vi "Autonomous Independent.vi"() -> ()   [LabVIEW 2016]
doc: "This VI is called when autonomous begins, and will automatically be terminated when autonomous ends. You can carry out timed or sensor driven robot movement independently without needing to return to the caller."
uses:
  <vilib>/Rock Robotics/WPI/Utilities/WPI_GetSetVariantRefNum.vi
  <vilib>/Rock Robotics/Network Tables/NT Write Numeric Array.vi
  <vilib>/Rock Robotics/Network Tables/NT Read Boolean.vi
  <vilib>/Rock Robotics/Network Tables/NT Write Number.vi
  <vilib>/Rock Robotics/WPI/RobotDrive/WPI_RobotDriveArcadeDrive_Standard(NoSaturation).vi
  <vilib>/Rock Robotics/Network Tables/NT Write Boolean.vi
  <vilib>/Rock Robotics/Network Tables/NT Read Number.vi
panel:
  out "Left + Right OverSpeed":cluster{dbl, dbl}(knob)={10.0, -10.0} scale=-10.0..10.0
  out "Difference":dbl(knob) scale=0.0..50.0
  in  "Reset Counters":bool
  out "Right Wheel Sensor Count":dbl
  out "Left Wheel Sensor Count":dbl
  out "POT Sensor Meter 3":dbl(knob)=78.0 scale=78.0..98.0
  out "POT Sensor Value 3":dbl
  out "Frame 0 - Hit Low Sensor":bool
  out "Frame 10 - Raised to Value":bool
  out "Frame 8  - TickSensor 1":bool
  out "Frame 6  - TickSensor 1":bool
  out "Frame 4 - TickSensor 1":bool
  out "Frame 2 - TickSensor 1":bool
  in  "Ticks to Turn Right":i32
  in  "To goto the edge of the goal":i32=9
  in  "Value to Raise to.":dbl=90.0
  in  "Ticks to Turn Left":i32=9
  in  "Distance to goto pass the Defence":i32=30
  in  "Ticks to Drive forwad close to the turnning Point":i32=42
  in  "Desides the Distance for Loop 1":i32=16
  out "VAR-Storage-1":dbl
  out "Low Switch":bool
  out "High Switch":bool
  # "Also This value is the \nTotal amount of ticks not Turns!\n\nSo 6 Ticks EQU 1 Full Turn."
  # "Remeber to Right Click:\nData Operatoins -> Make Current Value Default"
  # "LOOP 1 - LOOP 1 - LOOP 1 - LOOP 1 - LOOP 1 - LOOP 1 - LOOP 1 - LOOP 1 - LOOP 1 - LOOP 1 - LOOP 1"
  # "DRIVE PAST THE DEFENCE"
  # "LOOP 2  - LOOP 2  - LOOP 2  - LOOP 2  - LOOP 2  - LOOP 2 -  LOOP 2 - LOOP 2  - LOOP 2  - LOOP 2 - LOOP 2"
  # "THIS IS TO DRIVE PAST THE DEFENCE AND TRY TO SHOT"
  # "Left"
  # "Right"
  # "LOOP 3  - LOOP 3  - LOOP 3  - LOOP 3  - LOOP 3  - LOOP 3  - LOOP 3  - LOOP 3  - LOOP 3  - LOOP 3 - LOOP 3"
  # "Go Past the Defence."
  # "Be sure to right-click and choose Data Operations>>Make Current Value default if you want to save the array values with the VI"
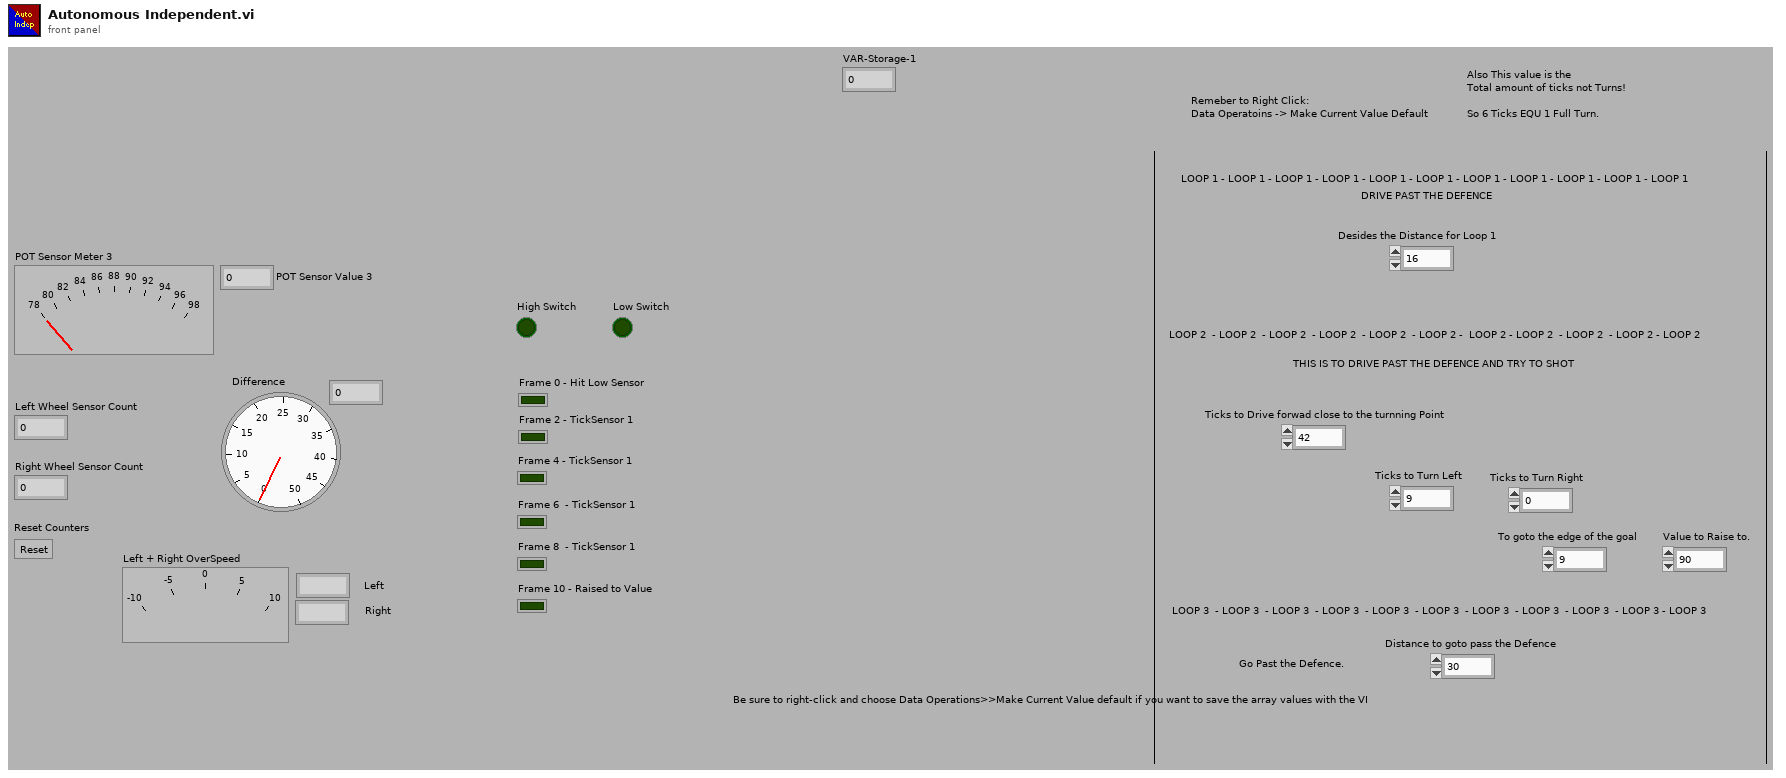
[diagram p1: front panel]
types:
  T1 = typedef "WPI_JoystickDevRef.ctl" = cluster{"Device":T2}
  T2 = typedef "WPI_JoystickDeviceEnum.ctl" = enum16{"USB 0", "USB 1", "USB 2", "USB 3", "USB 4", "USB 5"}
  T3 = typedef "WPI_RobotDriveDevRef.ctl" = cluster{"DevStatus":errorcluster, "Motors[]":T4[], "Square Inputs":bool, "Max Output":dbl}
  T4 = typedef "WPI_MotorControlDeviceRef.ctl" = cluster{"DeviceStatus":errorcluster, "Type":T5, "PWM":cluster{"PWM Channel":T6, "DeadBand":T7}, "CAN":cluster{"Device Number":u8, "SetOutput VI Ref":variant, "GetOutput VI Ref":variant, "Enable VI Ref":variant, "Disable VI Ref":variant, "Data":variant}, "Invert":bool}
  T5 = typedef "WPI_MotorControlType.ctl" = enum16{"PWM", "CAN"}
  T6 = typedef "FPGA_DIOPWMChannel.ctl" = enum8{"PWM 0", "PWM 1", "PWM 2", "PWM 3", "PWM 4", "PWM 5", "PWM 6", "PWM 7", "PWM 8", "PWM 9", "PWM MXP 0", "PWM MXP 1", "PWM MXP 2", "PWM MXP 3", "PWM MXP 4", "PWM MXP 5", "PWM MXP 6", "PWM MXP 7", "PWM MXP 8", "PWM MXP 9", "Invalid"}
  T7 = typedef "WPI_PWMDeadband.ctl" = cluster{"Name":string, "maxPositivePwm":i32, "minPositivePwm":i32, "centerPwm":i32, "maxNegativePwm":i32, "minNegativePwm":i32, "angularRange":u16}
  T8 = typedef "WPI_CounterDevRef.ctl" = cluster{"DevStatus":errorcluster, "CntIndex":T9}
  T9 = typedef "FPGA_CounterCtrSystemIndex.ctl" = enum8{"Ctr 0", "Ctr 1", "Ctr 2", "Ctr 3", "Ctr 4", "Ctr 5", "Ctr 6", "Ctr 7", "Invalid"}
  T10 = typedef "WPI_SwitchDevRef.ctl" = cluster{"DevStatus":errorcluster, "DIO Channel":T11, "CntIndex":T9, "Normally Closed":bool}
  T11 = typedef "FPGA_DIOChannel.ctl" = enum8{"DIO 0", "DIO 1", "DIO 2", "DIO 3", "DIO 4", "DIO 5", "DIO 6", "DIO 7", "DIO 8", "DIO 9", "DIO MXP 0", "DIO MXP 1", "DIO MXP 2", "DIO MXP 3", "DIO MXP 4", "DIO MXP 5", "DIO MXP 6", "DIO MXP 7", "DIO MXP 8", "DIO MXP 9", "DIO MXP 10", "DIO MXP 11", "DIO MXP 12", "DIO MXP 13", "DIO MXP 14", "DIO MXP 15", "SPI Port CS1", "SPI Port CS2", "SPI Port CS3", "SPI Port MISO", "SPI Port MOSI", "Invalid"}
  T12 = typedef "WPI_PotentiometerDevRef.ctl" = cluster{"DevStatus":errorcluster, "Analog Channel":T13, "Invert Output":bool}
  T13 = typedef "FPGA_AIChannel.ctl" = enum8{"AI 0", "AI 1", "AI 2", "AI 3", "AI MXP 0", "AI MXP 1", "AI MXP 2", "AI MXP 3", "Invalid"}
  T14 = typedef "WPI_ServoDeviceRef.ctl" = cluster{"DeviceStatus":errorcluster, "PWM Channel":T6, "DeadBand":T7}
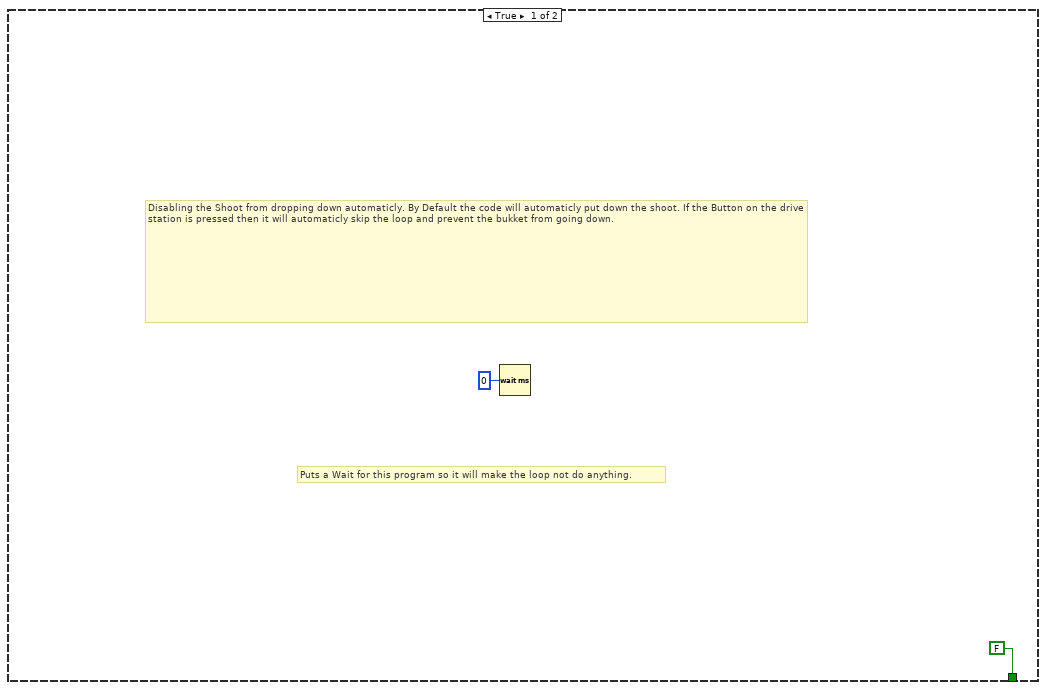
[diagram p3: hidden frame]
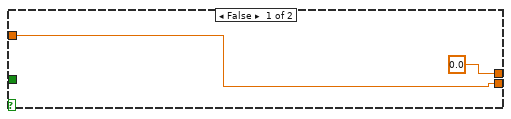
[diagram p4: hidden frame]
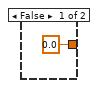
[diagram p5: hidden frame]
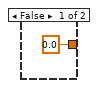
[diagram p7: hidden frame]
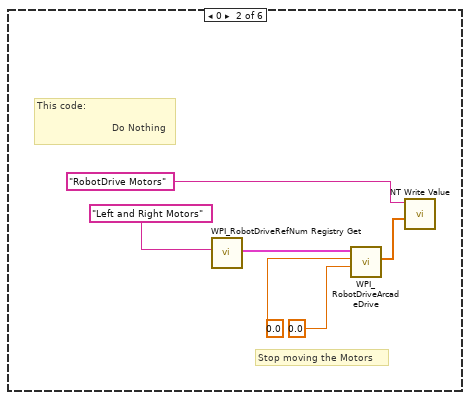
[diagram p10: hidden frame]
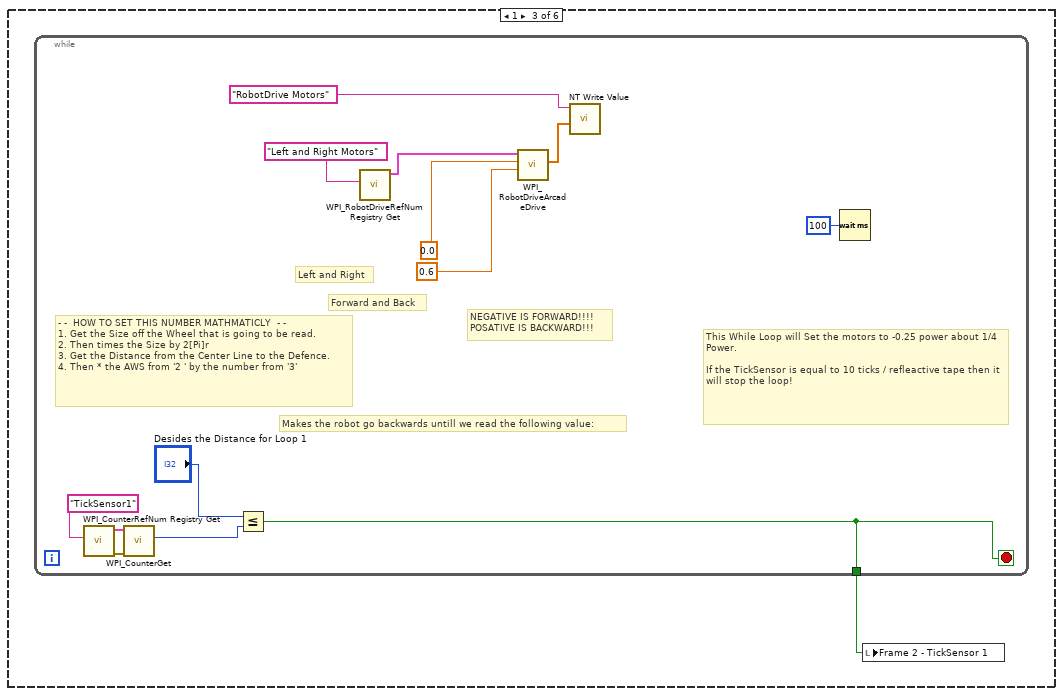
[diagram p11: hidden frame]
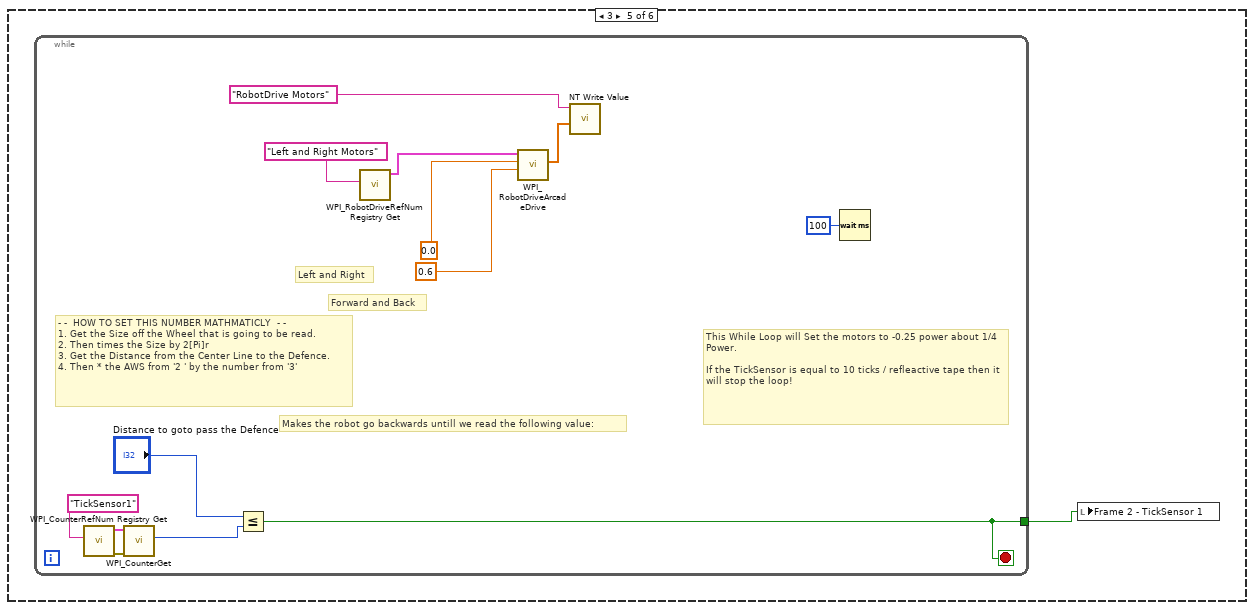
[diagram p12: hidden frame]
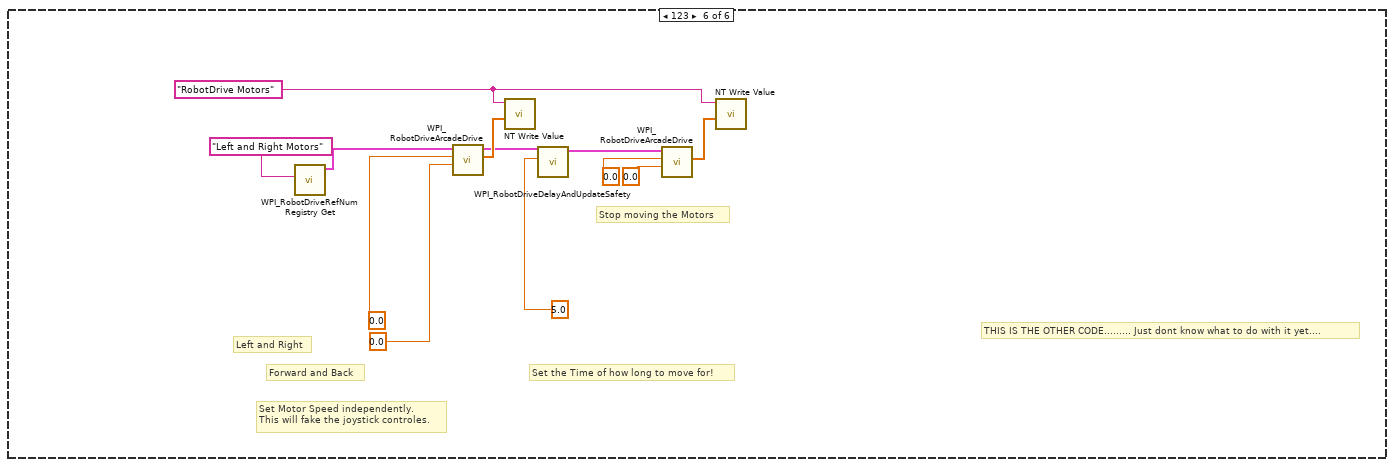
[diagram p13: hidden frame]
diagram:
  (unwired) "This function is run in parallel when the autonomous period begins. It will be terminated automatically when the period ends.\n\nNote that all Driver Station inputs are automatically latched and will not change once auto begins."
  # "Auto Count of Wheel"
  # "Every 20ms, report that we are running autonomous\ncode. Loop will abort the same time as the VI."
  # "This gives you the joystick value\nthat is often the throttle"
  # "This tells you the driver position\nand alliance color"
  n1 = call-poly <vilib>:"NT Read Value.vi"("Name"="Auto Selector") -> ()  [unwired: 9 in, 2 out]
  n2 = while {
    stop <- FALSE stop-if-true
    n3 = call <vilib>:"WPI_DriverStationReport Robot Code State.vi"("Autonomous"=TRUE) -> ()  [unwired: 10 in, 1 out]
    n4 = Wait (ms)(milliseconds to wait=u32 20) -> ()  [unwired: 1 out]
  }
  n5 = call <vilib>:"WPI_JoystickRefNum Registry Get.vi"("refnum name"="Joystick 0") -> ("JoystickDevRef"=w24:T1)  [unwired: 1 in, 9 out]
  n6 = call <vilib>:"WPI_JoystickGetValues.vi"("JoystickDevRef"=w24) -> ("Axes"=w22:dbl[])  [unwired: 6 in, 4 out]
  n7 = call <vilib>:"WPI_DriverStationGet Alliance Info.vi"() -> ()  [unwired: 12 out]
  n8 = call-poly <vilib>:"NT Write Value.vi"("Numeric Array"=w22, "Name"="Joystick 0/Axes") -> ()  [unwired: 9 in, 1 out]
  n9 = Index Array(array=w22, index=2) -> ()  [unwired: 1 out]
  n10 = flat-sequence {
    frame #0 {
      n11 = call <vilib>:"WPI_RobotDriveRefNum Registry Get.vi"("refnum name"="Left and Right Motors") -> ("RobotDriveDevRef"=w36:T3)  [unwired: 1 in, 9 out]
      n12 = call <vilib>:"WPI_MotorControlRefNum Registry Get.vi"("refnum name"="BPMs") -> ("error out"=w31:errorcluster, "MotorControlDevRef"=w30:T4)  [unwired: 9 in]
      n13 = call <vilib>:"WPI_CounterRefNum Registry Get.vi"("refnum name"="TickSensor1") -> ("error out"=w34:errorcluster, "CounterDevRef"=w35:T8)  [unwired: 9 in]
      n14 = call <vilib>:"WPI_CounterRefNum Registry Get.vi"("refnum name"="TickSensor2") -> ("error out"=w43:errorcluster, "CounterDevRef"=w42:T8)  [unwired: 9 in]
      n15 = call <vilib>:"WPI_CounterReset.vi"("error in (no error)"=w34, "CounterDevRef in"=w35) -> ()  [unwired: 8 in, 2 out]
      n16 = call <vilib>:"WPI_CounterReset.vi"("error in (no error)"=w43, "CounterDevRef in"=w42) -> ()  [unwired: 8 in, 2 out]
      n17 = call <vilib>:"WPI_MotorControlSetOutput.vi"("error in (no error)"=w31, "Output"=0.0, "MotorControlDevRef"=w30) -> ()  [unwired: 6 in, 3 out]
      n18 = call-poly <vilib>:"WPI_RobotDriveArcadeDrive.vi"("Y axis value"=0.0 ("X axis value"), "X axis value"=0.0, "RobotDriveDevRef"=w36) -> ("Motor Values"=w38:dbl[])  [unwired: 1 in, 7 out]
      n19 = call-poly <vilib>:"NT Write Value.vi"("Numeric Array"=w38, "Name"="RobotDrive Motors") -> ()  [unwired: 9 in, 1 out]
    }
    frame #1 {
      n20 = call-poly <vilib>:"NT Read Value.vi"("Default Value"=FALSE, "Name"="DisableLowerOnStart") -> ()  [unwired: 8 in, 2 out]
      n21 = case shown="False" FALSE {
        tunnel: [FALSE w51] -> w45
        frame True {
          # "Puts a Wait for this program so it will make the loop not do anything."
          # "Disabling the Shoot from dropping down automaticly. By Default the code will automaticly put down the shoot. If the Button on the drive station is pressed then it will automaticly skip the loop and prevent the bukket from going down."
          n22 = Wait (ms)(milliseconds to wait=u32 0) -> ()  [unwired: 1 out]
        }
        frame False {
          n23 = while {
            tunnel: [w52] -> w51
            stop <- w52 stop-if-true
            n24 = call <vilib>:"WPI_SwitchRefNum Registry Get.vi"("refnum name"="LowSwitch") -> ("error out"=w69:errorcluster, "SwitchDevRef"=w70:T10)  [unwired: 9 in]
            n25 = call <vilib>:"WPI_SwitchRefNum Registry Get.vi"("refnum name"="HighSwitch") -> ("error out"=w66:errorcluster, "SwitchDevRef"=w67:T10)  [unwired: 9 in]
            n26 = call <vilib>:"WPI_SwitchGetLimitValue.vi"("error in (no error)"=w69, "SwitchDevRef"=w70) -> ("Switch Pressed"=w58:bool)  [unwired: 7 in, 2 out]
            "Low Switch" <- w58
            n27 = call <vilib>:"WPI_SwitchGetLimitValue.vi"("error in (no error)"=w66, "SwitchDevRef"=w67) -> ("Switch Pressed"=w57:bool)  [unwired: 7 in, 2 out]
            "High Switch" <- w57
            n28 = call-poly <vilib>:"NT Write Value.vi"("Boolean"=w58, "Name"="Low Sensor") -> ()  [unwired: 9 in, 1 out]
            n29 = call-poly <vilib>:"NT Write Value.vi"("Boolean"=w57, "Name"="High Sensor") -> ()  [unwired: 9 in, 1 out]
            n30 = Or(x=w58, y=w57) -> (x .or. y?=w71:bool)
            n31 = case shown="True" w71 {
              tunnel: w58 -> [_ w76]
              tunnel: w57 -> [_ w78]
              tunnel: -0.5 ("Axes[1]") -> [w72 w77]
              tunnel: [0.0 ("Axes[1]") w75] -> w60
              tunnel: [w72 w74] -> w59
              frame False {
              }
              frame True {
                n32 = case shown="True" w76 {
                  tunnel: w77 -> [_ w88]
                  tunnel: [0.0 ("Axes[1]") w87] -> w75
                  frame False {
                  }
                  frame True {
                    n33 = Greater?(x=w88, y=0.0) -> (0:w89:bool)
                    n34 = case shown="False" w89 {
                      tunnel: [0.0 ("Axes[1]") w92] -> w87
                      tunnel: w88 -> [_ w92]
                      frame False {
                        # "NO VALUE SENT"
                      }
                      frame True {
                      }
                    }
                  }
                }
                n35 = case shown="True" w78 {
                  tunnel: w77 -> [_ w80]
                  tunnel: [0.0 ("Axes[1]") w81] -> w74
                  frame False {
                  }
                  frame True {
                    n36 = Less?(x=w80, y=0.0) -> (x < y?=w82:bool)
                    n37 = case shown="False" w82 {
                      tunnel: [0.0 ("Axes[1]") w85] -> w81
                      tunnel: w80 -> [_ w85]
                      frame False {
                        # "NO VALUE SENT"
                      }
                      frame True {
                      }
                    }
                  }
                }
              }
            }
            n38 = Add(x=w60, y=w59) -> (x+y=w61:dbl)
            n39 = call <vilib>:"WPI_MotorControlRefNum Registry Get.vi"("refnum name"="Pickup Motor") -> ("error out"=w64:errorcluster, "MotorControlDevRef"=w63:T4)  [unwired: 9 in]
            n40 = local read "Low Switch"() -> (w52:bool)
            n41 = call <vilib>:"WPI_MotorControlSetOutput.vi"("error in (no error)"=w64, "Output"=w61, "MotorControlDevRef"=w63) -> ()  [unwired: 6 in, 3 out]
            n42 = Wait (ms)(milliseconds to wait=u32 100) -> ()  [unwired: 1 out]
          }
        }
      }
      "Frame 0 - Hit Low Sensor" <- w45
    }
    frame #2 {
      # "This tells you the autonomous selected\nfrom the dashboard"
      n43 = call-poly <vilib>:"NT Read Value.vi"("Name"="AutoModeSelector") -> ("Numeric"=w94:dbl)  [unwired: 9 in, 1 out]
      n44 = Wait (ms)(milliseconds to wait=u32 20) -> ()  [unwired: 1 out]
      n45 = case shown="2" w94 {
        frame Default {
          # "You can put your main auto here, or you can right-click on the case and make any\nother frame be the default case."
          # "This is the frame that will execute if no selection is made, or if it is not recognized"
        }
        frame 0 {
          # "Stop moving the Motors"
          # "This code:\n                   \n                         Do Nothing"
          n46 = call <vilib>:"WPI_RobotDriveRefNum Registry Get.vi"("refnum name"="Left and Right Motors") -> ("RobotDriveDevRef"=w96:T3)  [unwired: 1 in, 9 out]
          n47 = call-poly <vilib>:"WPI_RobotDriveArcadeDrive.vi"("Y axis value"=0.0 ("X axis value"), "X axis value"=0.0, "RobotDriveDevRef"=w96) -> ("Motor Values"=w100:dbl[])  [unwired: 1 in, 7 out]
          n48 = call-poly <vilib>:"NT Write Value.vi"("Numeric Array"=w100, "Name"="RobotDrive Motors") -> ()  [unwired: 9 in, 1 out]
        }
        frame 1 {
          n49 = while {
            tunnel: [w103] -> w102
            stop <- w103 stop-if-true
            # "NEGATIVE IS FORWARD!!!!\nPOSATIVE IS BACKWARD!!!"
            # "- -  HOW TO SET THIS NUMBER MATHMATICLY  - - \n1. Get the Size off the Wheel that is going to be read.\n2. Then times the Size by 2[Pi]r\n3. Get the Distance from the Center Line to the Defence.\n4. Then * the AWS from '2 ' by the number from '3'"
            # "Makes the robot go backwards untill we read the following value:"
            # "This While Loop will Set the motors to -0.25 power about 1/4 Power.\n\nIf the TickSensor is equal to 10 ticks / refleactive tape then it will stop the loop!"
            # "Forward and Back"
            # "Left and Right"
            n50 = call <vilib>:"WPI_CounterRefNum Registry Get.vi"("refnum name"="TickSensor1") -> ("error out"=w114:errorcluster, "CounterDevRef"=w113:T8)  [unwired: 9 in]
            n51 = call <vilib>:"WPI_CounterGet.vi"("error in (no error)"=w114, "CounterDevRef in"=w113) -> ("Value"=w105:i32)  [unwired: 4 in, 5 out]
            n52 = Less Or Equal?(x="Desides the Distance for Loop 1", y=w105) -> (x <= y?=w103:bool)
            n53 = call <vilib>:"WPI_RobotDriveRefNum Registry Get.vi"("refnum name"="Left and Right Motors") -> ("RobotDriveDevRef"=w112:T3)  [unwired: 1 in, 9 out]
            n54 = call-poly <vilib>:"WPI_RobotDriveArcadeDrive.vi"("Y axis value"=0.6 ("X axis value"), "X axis value"=0.0, "RobotDriveDevRef"=w112) -> ("Motor Values"=w110:dbl[])  [unwired: 1 in, 7 out]
            n55 = call-poly <vilib>:"NT Write Value.vi"("Numeric Array"=w110, "Name"="RobotDrive Motors") -> ()  [unwired: 9 in, 1 out]
            n56 = Wait (ms)(milliseconds to wait=u32 100) -> ()  [unwired: 1 out]
          }
          n57 = local write "Frame 2 - TickSensor 1"(w102) -> ()
        }
        frame 2 {
          n58 = flat-sequence {
            frame #0 {
              n59 = while {
                tunnel: [w117] -> w116
                stop <- w117 stop-if-true
                # "- -  HOW TO SET THIS NUMBER MATHMATICLY  - - \n1. Get the Size off the Wheel that is going to be read.\n2. Then times the Size by 2[Pi]r\n3. Get the Distance from the Center Line to the Defence.\n4. Then * the AWS from '2 ' by the number from '3'"
                # "Makes the robot go backwards untill we read the following value:"
                # "This While Loop will Set the motors to -0.25 power about 1/4 Power.\n\nIf the TickSensor is equal to 10 ticks / refleactive tape then it will stop the loop!"
                # "Forward and Back"
                # "Left and Right"
                n60 = call <vilib>:"WPI_CounterRefNum Registry Get.vi"("refnum name"="TickSensor1") -> ("error out"=w128:errorcluster, "CounterDevRef"=w127:T8)  [unwired: 9 in]
                n61 = Wait (ms)(milliseconds to wait=u32 100) -> ()  [unwired: 1 out]
                n62 = call <vilib>:"WPI_CounterGet.vi"("error in (no error)"=w128, "CounterDevRef in"=w127) -> ("Value"=w119:i32)  [unwired: 4 in, 5 out]
                n63 = Less Or Equal?(x="Ticks to Drive forwad close to the turnning Point", y=w119) -> (x <= y?=w117:bool)
                n64 = call <vilib>:"WPI_RobotDriveRefNum Registry Get.vi"("refnum name"="Left and Right Motors") -> ("RobotDriveDevRef"=w126:T3)  [unwired: 1 in, 9 out]
                n65 = call-poly <vilib>:"WPI_RobotDriveArcadeDrive.vi"("Y axis value"=0.6 ("X axis value"), "X axis value"=0.0, "RobotDriveDevRef"=w126) -> ("Motor Values"=w124:dbl[])  [unwired: 1 in, 7 out]
                n66 = call-poly <vilib>:"NT Write Value.vi"("Numeric Array"=w124, "Name"="RobotDrive Motors") -> ()  [unwired: 9 in, 1 out]
              }
              "Frame 2 - TickSensor 1" <- w116
            }
            frame #1 {
              n67 = call <vilib>:"WPI_CounterRefNum Registry Get.vi"("refnum name"="TickSensor2") -> ("error out"=w137:errorcluster, "CounterDevRef"=w136:T8)  [unwired: 9 in]
              n68 = call <vilib>:"WPI_RobotDriveRefNum Registry Get.vi"("refnum name"="Left and Right Motors") -> ("RobotDriveDevRef"=w135:T3)  [unwired: 1 in, 9 out]
              n69 = call-poly <vilib>:"WPI_RobotDriveArcadeDrive.vi"("Y axis value"=0.0 ("X axis value"), "X axis value"=0.0, "RobotDriveDevRef"=w135) -> ("Motor Values"=w133:dbl[])  [unwired: 1 in, 7 out]
              n70 = call <vilib>:"WPI_CounterRefNum Registry Get.vi"("refnum name"="TickSensor1") -> ("error out"=w140:errorcluster, "CounterDevRef"=w139:T8)  [unwired: 9 in]
              n71 = call <vilib>:"WPI_CounterReset.vi"("error in (no error)"=w137, "CounterDevRef in"=w136) -> ()  [unwired: 8 in, 2 out]
              n72 = call <vilib>:"WPI_CounterReset.vi"("error in (no error)"=w140, "CounterDevRef in"=w139) -> ()  [unwired: 8 in, 2 out]
              n73 = call-poly <vilib>:"NT Write Value.vi"("Numeric Array"=w133, "Name"="RobotDrive Motors") -> ()  [unwired: 9 in, 1 out]
            }
            frame #2 {
              n74 = while {
                tunnel: [w144] -> w142
                stop <- w144 stop-if-true
                # "Forward and Back"
                # "Left and Right"
                n75 = call <vilib>:"WPI_CounterRefNum Registry Get.vi"("refnum name"="TickSensor1") -> ("error out"=w154:errorcluster, "CounterDevRef"=w153:T8)  [unwired: 9 in]
                n76 = call <vilib>:"WPI_CounterGet.vi"("error in (no error)"=w154, "CounterDevRef in"=w153) -> ("Value"=w147:i32)  [unwired: 4 in, 5 out]
                n77 = call <vilib>:"WPI_RobotDriveRefNum Registry Get.vi"("refnum name"="Left and Right Motors") -> ("RobotDriveDevRef"=w152:T3)  [unwired: 1 in, 9 out]
                n78 = Less Or Equal?(x="Ticks to Turn Left", y=w147) -> (x <= y?=w144:bool)
                n79 = call-poly <vilib>:"WPI_RobotDriveArcadeDrive.vi"("Y axis value"=0.0 ("X axis value"), "X axis value"=-0.5, "RobotDriveDevRef"=w152) -> ("Motor Values"=w151:dbl[])  [unwired: 1 in, 7 out]
                n80 = call-poly <vilib>:"NT Write Value.vi"("Numeric Array"=w151, "Name"="RobotDrive Motors") -> ()  [unwired: 9 in, 1 out]
              }
              "Frame 4 - TickSensor 1" <- w142
              n81 = Wait (ms)(milliseconds to wait=u32 100) -> ()  [unwired: 1 out]
            }
            frame #3 {
              n82 = call <vilib>:"WPI_RobotDriveRefNum Registry Get.vi"("refnum name"="Left and Right Motors") -> ("RobotDriveDevRef"=w156:T3)  [unwired: 1 in, 9 out]
              n83 = call-poly <vilib>:"WPI_RobotDriveArcadeDrive.vi"("Y axis value"=0.0 ("X axis value"), "X axis value"=0.0, "RobotDriveDevRef"=w156) -> ("Motor Values"=w158:dbl[])  [unwired: 1 in, 7 out]
              n84 = call-poly <vilib>:"NT Write Value.vi"("Numeric Array"=w158, "Name"="RobotDrive Motors") -> ()  [unwired: 9 in, 1 out]
            }
            frame #4 {
              n85 = while {
                tunnel: [w164] -> w162
                stop <- w164 stop-if-true
                # "Forward and Back"
                # "Left and Right"
                n86 = call <vilib>:"WPI_CounterRefNum Registry Get.vi"("refnum name"="TickSensor2") -> ("error out"=w174:errorcluster, "CounterDevRef"=w173:T8)  [unwired: 9 in]
                n87 = call <vilib>:"WPI_RobotDriveRefNum Registry Get.vi"("refnum name"="Left and Right Motors") -> ("RobotDriveDevRef"=w172:T3)  [unwired: 1 in, 9 out]
                n88 = call <vilib>:"WPI_CounterGet.vi"("error in (no error)"=w174, "CounterDevRef in"=w173) -> ("Value"=w167:i32)  [unwired: 4 in, 5 out]
                n89 = call-poly <vilib>:"WPI_RobotDriveArcadeDrive.vi"("Y axis value"=0.0 ("X axis value"), "X axis value"=0.5, "RobotDriveDevRef"=w172) -> ("Motor Values"=w171:dbl[])  [unwired: 1 in, 7 out]
                n90 = Less Or Equal?(x="Ticks to Turn Right", y=w167) -> (x <= y?=w164:bool)
                n91 = call-poly <vilib>:"NT Write Value.vi"("Numeric Array"=w171, "Name"="RobotDrive Motors") -> ()  [unwired: 9 in, 1 out]
              }
              "Frame 6  - TickSensor 1" <- w162
              n92 = Wait (ms)(milliseconds to wait=u32 100) -> ()  [unwired: 1 out]
            }
            frame #5 {
              n93 = call <vilib>:"WPI_CounterRefNum Registry Get.vi"("refnum name"="TickSensor2") -> ("error out"=w183:errorcluster, "CounterDevRef"=w182:T8)  [unwired: 9 in]
              n94 = call <vilib>:"WPI_CounterRefNum Registry Get.vi"("refnum name"="TickSensor1") -> ("error out"=w186:errorcluster, "CounterDevRef"=w185:T8)  [unwired: 9 in]
              n95 = call <vilib>:"WPI_RobotDriveRefNum Registry Get.vi"("refnum name"="Left and Right Motors") -> ("RobotDriveDevRef"=w181:T3)  [unwired: 1 in, 9 out]
              n96 = call-poly <vilib>:"WPI_RobotDriveArcadeDrive.vi"("Y axis value"=0.0 ("X axis value"), "X axis value"=0.0, "RobotDriveDevRef"=w181) -> ("Motor Values"=w179:dbl[])  [unwired: 1 in, 7 out]
              n97 = call <vilib>:"WPI_CounterReset.vi"("error in (no error)"=w183, "CounterDevRef in"=w182) -> ()  [unwired: 8 in, 2 out]
              n98 = call <vilib>:"WPI_CounterReset.vi"("error in (no error)"=w186, "CounterDevRef in"=w185) -> ()  [unwired: 8 in, 2 out]
              n99 = call-poly <vilib>:"NT Write Value.vi"("Numeric Array"=w179, "Name"="RobotDrive Motors") -> ()  [unwired: 9 in, 1 out]
            }
            frame #6 {
              n100 = while {
                tunnel: [w189] -> w188
                stop <- w189 stop-if-true
                # "- -  HOW TO SET THIS NUMBER MATHMATICLY  - - \n1. Get the Size off the Wheel that is going to be read.\n2. Then times the Size by 2[Pi]r\n3. Get the Distance from the Center Line to the Defence.\n4. Then * the AWS from '2 ' by the number from '3'"
                # "Makes the robot go backwards untill we read the following value:"
                # "This While Loop will Set the motors to -0.25 power about 1/4 Power.\n\nIf the TickSensor is equal to 10 ticks / refleactive tape then it will stop the loop!"
                # "Forward and Back"
                # "Left and Right"
                n101 = call <vilib>:"WPI_CounterRefNum Registry Get.vi"("refnum name"="TickSensor1") -> ("error out"=w200:errorcluster, "CounterDevRef"=w199:T8)  [unwired: 9 in]
                n102 = Wait (ms)(milliseconds to wait=u32 100) -> ()  [unwired: 1 out]
                n103 = call <vilib>:"WPI_CounterGet.vi"("error in (no error)"=w200, "CounterDevRef in"=w199) -> ("Value"=w191:i32)  [unwired: 4 in, 5 out]
                n104 = Less Or Equal?(x="To goto the edge of the goal", y=w191) -> (x <= y?=w189:bool)
                n105 = call <vilib>:"WPI_RobotDriveRefNum Registry Get.vi"("refnum name"="Left and Right Motors") -> ("RobotDriveDevRef"=w198:T3)  [unwired: 1 in, 9 out]
                n106 = call-poly <vilib>:"WPI_RobotDriveArcadeDrive.vi"("Y axis value"=-0.6 ("X axis value"), "X axis value"=0.0, "RobotDriveDevRef"=w198) -> ("Motor Values"=w196:dbl[])  [unwired: 1 in, 7 out]
                n107 = call-poly <vilib>:"NT Write Value.vi"("Numeric Array"=w196, "Name"="RobotDrive Motors") -> ()  [unwired: 9 in, 1 out]
              }
              "Frame 8  - TickSensor 1" <- w188
            }
            frame #7 {
              n108 = call <vilib>:"WPI_CounterRefNum Registry Get.vi"("refnum name"="TickSensor2") -> ("error out"=w209:errorcluster, "CounterDevRef"=w208:T8)  [unwired: 9 in]
              n109 = call <vilib>:"WPI_CounterRefNum Registry Get.vi"("refnum name"="TickSensor1") -> ("error out"=w212:errorcluster, "CounterDevRef"=w211:T8)  [unwired: 9 in]
              n110 = call <vilib>:"WPI_CounterReset.vi"("error in (no error)"=w209, "CounterDevRef in"=w208) -> ()  [unwired: 8 in, 2 out]
              n111 = call <vilib>:"WPI_CounterReset.vi"("error in (no error)"=w212, "CounterDevRef in"=w211) -> ()  [unwired: 8 in, 2 out]
              n112 = call <vilib>:"WPI_RobotDriveRefNum Registry Get.vi"("refnum name"="Left and Right Motors") -> ("RobotDriveDevRef"=w207:T3)  [unwired: 1 in, 9 out]
              n113 = call-poly <vilib>:"WPI_RobotDriveArcadeDrive.vi"("Y axis value"=0.0 ("X axis value"), "X axis value"=0.0, "RobotDriveDevRef"=w207) -> ("Motor Values"=w205:dbl[])  [unwired: 1 in, 7 out]
              n114 = call-poly <vilib>:"NT Write Value.vi"("Numeric Array"=w205, "Name"="RobotDrive Motors") -> ()  [unwired: 9 in, 1 out]
            }
            frame #8 {
              n115 = call "Time Delay"("Delay Time (s)"=1.0) -> ()  [unwired: 10 in, 1 out]
            }
            frame #9 {
              n116 = while {
                tunnel: [w216] -> w215
                stop <- w216 stop-if-true
                # "This value will set the pickup motors to lift them up."
                # "This value will be the P.O.T. value. This will stop the Loop from running."
                n117 = call <vilib>:"WPI_PotentiometerRefNum Registry Get.vi"("refnum name"="POT Sensor") -> ("error out"=w228:errorcluster, "PotDevRef"=w227:T12)  [unwired: 9 in]
                n118 = call <vilib>:"WPI_PotentiometerGetNormalized.vi"("error in"=w228, "PotDevRef"=w227) -> ("Normalized Value"=w225:dbl)  [unwired: 7 in, 2 out]
                n119 = Multiply(x=w225, y=100.0) -> (x*y=w223:dbl)
                n120 = call <vilib>:"WPI_MotorControlRefNum Registry Get.vi"("refnum name"="Pickup Motor") -> ("error out"=w222:errorcluster, "MotorControlDevRef"=w221:T4)  [unwired: 9 in]
                n121 = Less Or Equal?(x=w223, y="Value to Raise to.") -> (x <= y?=w216:bool)
                n122 = call <vilib>:"WPI_MotorControlSetOutput.vi"("error in (no error)"=w222, "Output"=0.6, "MotorControlDevRef"=w221) -> ()  [unwired: 6 in, 3 out]
                n123 = Wait (ms)(milliseconds to wait=u32 100) -> ()  [unwired: 1 out]
              }
              "Frame 10 - Raised to Value" <- w215
            }
            frame #10 {
              n124 = call <vilib>:"WPI_MotorControlRefNum Registry Get.vi"("refnum name"="BPMs") -> ("error out"=w235:errorcluster, "MotorControlDevRef"=w234:T4)  [unwired: 9 in]
              n125 = call <vilib>:"WPI_MotorControlRefNum Registry Get.vi"("refnum name"="Pickup Motor") -> ("error out"=w231:errorcluster, "MotorControlDevRef"=w230:T4)  [unwired: 9 in]
              n126 = call <vilib>:"WPI_MotorControlSetOutput.vi"("error in (no error)"=w235, "Output"=0.0, "MotorControlDevRef"=w234) -> ()  [unwired: 6 in, 3 out]
              n127 = call <vilib>:"WPI_MotorControlSetOutput.vi"("error in (no error)"=w231, "Output"=0.0, "MotorControlDevRef"=w230) -> ()  [unwired: 6 in, 3 out]
            }
            frame #11 {
              n128 = call "Time Delay3"("Delay Time (s)"=0.5) -> ()  [unwired: 10 in, 1 out]
            }
            frame #12 {
              n129 = call <vilib>:"WPI_MotorControlRefNum Registry Get.vi"("refnum name"="BPMs") -> ("error out"=w240:errorcluster, "MotorControlDevRef"=w239:T4)  [unwired: 9 in]
              n130 = call <vilib>:"WPI_MotorControlSetOutput.vi"("error in (no error)"=w240, "Output"=-0.75, "MotorControlDevRef"=w239) -> ()  [unwired: 6 in, 3 out]
            }
            frame #13 {
              n131 = call "Time Delay2"("Delay Time (s)"=0.5) -> ()  [unwired: 10 in, 1 out]
            }
            frame #14 {
              # "Sets the Servo to TRUE so it goes to the full open position."
              # "The Low Value"
              n132 = Select(t=0.0, s=TRUE, f=0.3) -> (s? t:f=w244:dbl)
              n133 = call <vilib>:"WPI_ServoRefNum Registry Get.vi"("refnum name"="Servo 1") -> ("error out"=w248:errorcluster, "ServoDeviceRef"=w247:T14)  [unwired: 9 in]
              n134 = call <vilib>:"WPI_ServoSetPosition.vi"("error in (no error)"=w248, "Position"=w244, "ServoDeviceRef"=w247) -> ()  [unwired: 7 in, 2 out]
            }
          }
        }
        frame 3 {
          n135 = while {
            tunnel: [w251] -> w250
            stop <- w251 stop-if-true
            # "- -  HOW TO SET THIS NUMBER MATHMATICLY  - - \n1. Get the Size off the Wheel that is going to be read.\n2. Then times the Size by 2[Pi]r\n3. Get the Distance from the Center Line to the Defence.\n4. Then * the AWS from '2 ' by the number from '3'"
            # "Makes the robot go backwards untill we read the following value:"
            # "This While Loop will Set the motors to -0.25 power about 1/4 Power.\n\nIf the TickSensor is equal to 10 ticks / refleactive tape then it will stop the loop!"
            # "Forward and Back"
            # "Left and Right"
            n136 = call <vilib>:"WPI_CounterRefNum Registry Get.vi"("refnum name"="TickSensor1") -> ("error out"=w262:errorcluster, "CounterDevRef"=w261:T8)  [unwired: 9 in]
            n137 = call <vilib>:"WPI_CounterGet.vi"("error in (no error)"=w262, "CounterDevRef in"=w261) -> ("Value"=w253:i32)  [unwired: 4 in, 5 out]
            n138 = Less Or Equal?(x="Distance to goto pass the Defence", y=w253) -> (x <= y?=w251:bool)
            n139 = call <vilib>:"WPI_RobotDriveRefNum Registry Get.vi"("refnum name"="Left and Right Motors") -> ("RobotDriveDevRef"=w260:T3)  [unwired: 1 in, 9 out]
            n140 = call-poly <vilib>:"WPI_RobotDriveArcadeDrive.vi"("Y axis value"=0.6 ("X axis value"), "X axis value"=0.0, "RobotDriveDevRef"=w260) -> ("Motor Values"=w258:dbl[])  [unwired: 1 in, 7 out]
            n141 = call-poly <vilib>:"NT Write Value.vi"("Numeric Array"=w258, "Name"="RobotDrive Motors") -> ()  [unwired: 9 in, 1 out]
            n142 = Wait (ms)(milliseconds to wait=u32 100) -> ()  [unwired: 1 out]
          }
          n143 = local write "Frame 2 - TickSensor 1"(w250) -> ()
        }
        frame 123 {
          w274 = "RobotDrive Motors" ("Name")
          # "THIS IS THE OTHER CODE......... Just dont know what to do with it yet...."
          # "Forward and Back"
          # "Left and Right"
          # "Set Motor Speed independently.\nThis will fake the joystick controles."
          # "Set the Time of how long to move for!"
          # "Stop moving the Motors"
          n144 = call <vilib>:"WPI_RobotDriveRefNum Registry Get.vi"("refnum name"="Left and Right Motors") -> ("RobotDriveDevRef"=w275:T3)  [unwired: 1 in, 9 out]
          n145 = call-poly <vilib>:"WPI_RobotDriveArcadeDrive.vi"("Y axis value"=0.0 ("X axis value"), "X axis value"=0.0, "RobotDriveDevRef"=w275) -> ("Motor Values"=w273:dbl[], "RobotDriveDevRef"=w267:T3)  [unwired: 1 in, 6 out]
          n146 = call-poly <vilib>:"NT Write Value.vi"("Numeric Array"=w273, "Name"=w274) -> ()  [unwired: 9 in, 1 out]
          n147 = call <vilib>:"WPI_RobotDriveDelayAndUpdateSafety.vi"("Delay (s)"=5.0, "RobotDriveDevRef"=w267) -> ("RobotDriveDevRef 2"=w266:T3)  [unwired: 8 in, 1 out]
          n148 = call-poly <vilib>:"WPI_RobotDriveArcadeDrive.vi"("Y axis value"=0.0 ("X axis value"), "X axis value"=0.0, "RobotDriveDevRef"=w266) -> ("Motor Values"=w272:dbl[])  [unwired: 1 in, 7 out]
          n149 = call-poly <vilib>:"NT Write Value.vi"("Numeric Array"=w272, "Name"=w274) -> ()  [unwired: 9 in, 1 out]
        }
      }
    }
    frame #3 {
      n150 = call <vilib>:"WPI_RobotDriveRefNum Registry Get.vi"("refnum name"="Left and Right Motors") -> ("RobotDriveDevRef"=w286:T3)  [unwired: 1 in, 9 out]
      n151 = call <vilib>:"WPI_MotorControlRefNum Registry Get.vi"("refnum name"="BPMs") -> ("error out"=w278:errorcluster, "MotorControlDevRef"=w277:T4)  [unwired: 9 in]
      n152 = call <vilib>:"WPI_CounterRefNum Registry Get.vi"("refnum name"="TickSensor2") -> ("error out"=w284:errorcluster, "CounterDevRef"=w285:T8)  [unwired: 9 in]
      n153 = call <vilib>:"WPI_CounterRefNum Registry Get.vi"("refnum name"="TickSensor1") -> ("error out"=w281:errorcluster, "CounterDevRef"=w282:T8)  [unwired: 9 in]
      n154 = call <vilib>:"WPI_MotorControlSetOutput.vi"("error in (no error)"=w278, "Output"=0.0, "MotorControlDevRef"=w277) -> ()  [unwired: 6 in, 3 out]
      n155 = call <vilib>:"WPI_CounterReset.vi"("error in (no error)"=w284, "CounterDevRef in"=w285) -> ()  [unwired: 8 in, 2 out]
      n156 = call <vilib>:"WPI_CounterReset.vi"("error in (no error)"=w281, "CounterDevRef in"=w282) -> ()  [unwired: 8 in, 2 out]
      n157 = call-poly <vilib>:"WPI_RobotDriveArcadeDrive.vi"("Y axis value"=0.0 ("X axis value"), "X axis value"=0.0, "RobotDriveDevRef"=w286) -> ("Motor Values"=w288:dbl[])  [unwired: 1 in, 7 out]
      n158 = call-poly <vilib>:"NT Write Value.vi"("Numeric Array"=w288, "Name"="RobotDrive Motors") -> ()  [unwired: 9 in, 1 out]
    }
  }
  n159 = call <vilib>:"WPI_PotentiometerRefNum Registry Get.vi"("refnum name"="POT Sensor") -> ("error out"=w19:errorcluster, "PotDevRef"=w18:T12)  [unwired: 9 in]
  n160 = call <vilib>:"WPI_PotentiometerGetNormalized.vi"("error in"=w19, "PotDevRef"=w18) -> ("Normalized Value"=w15:dbl)  [unwired: 7 in, 2 out]
  n161 = Multiply(x=w15, y=100.0) -> (x*y=w13:dbl)
  "POT Sensor Value 3" <- w13
  "POT Sensor Meter 3" <- w13
  n162 = call-poly <vilib>:"NT Write Value.vi"("Numeric"=w13, "Name"="POT Sensor") -> ()  [unwired: 9 in, 1 out]
  n163 = case shown="True" "Reset Counters" {
    frame False {
    }
    frame True {
      n164 = call <vilib>:"WPI_CounterRefNum Registry Get.vi"("refnum name"="TickSensor2") -> ("error out"=w296:errorcluster, "CounterDevRef"=w297:T8)  [unwired: 9 in]
      n165 = call <vilib>:"WPI_CounterRefNum Registry Get.vi"("refnum name"="TickSensor1") -> ("error out"=w293:errorcluster, "CounterDevRef"=w294:T8)  [unwired: 9 in]
      n166 = call <vilib>:"WPI_CounterReset.vi"("error in (no error)"=w296, "CounterDevRef in"=w297) -> ()  [unwired: 8 in, 2 out]
      n167 = call <vilib>:"WPI_CounterReset.vi"("error in (no error)"=w293, "CounterDevRef in"=w294) -> ()  [unwired: 8 in, 2 out]
    }
  }
  n168 = call <vilib>:"WPI_CounterRefNum Registry Get.vi"("refnum name"="TickSensor2") -> ("CounterDevRef"=w9:T8)  [unwired: 9 in, 1 out]
  n169 = call <vilib>:"WPI_CounterRefNum Registry Get.vi"("refnum name"="TickSensor1") -> ("CounterDevRef"=w11:T8)  [unwired: 9 in, 1 out]
  n170 = call <vilib>:"WPI_CounterGet.vi"("CounterDevRef in"=w9) -> ("Value"=w1:i32)  [unwired: 5 in, 5 out]
  "Right Wheel Sensor Count" <- w1
  n171 = call <vilib>:"WPI_CounterGet.vi"("CounterDevRef in"=w11) -> ("Value"=w2:i32)  [unwired: 5 in, 5 out]
  "Left Wheel Sensor Count" <- w2
  n172 = Subtract(x=w2, y=w1) -> (x-y=w4:i32)
  n173 = Subtract(x=w1, y=w2) -> (x-y=w3:i32)
  n174 = Bundle(w4, w3) -> (→"Left + Right OverSpeed":cluster{i32, i32})  [unwired: 1 in]
  n175 = Subtract(x=w2, y=w1) -> (x-y=w7:i32)
  n176 = Absolute Value(x=w7) -> (abs(x)=→"Difference":i32)
